vi "Stereo - Analyze Calibrated Image.vi"(8 "error in (no error)":errorcluster, 10 "Grid Images in":T4(array[cluster]), 11 "Calibrated Images in":T1[](array[typedef])) -> (0 "error out":errorcluster, 1 "Calibration OK":bool, 2 "Grid Images out":T4(array[cluster]), 3 "Calibrated Images out":T1[](array[typedef]))   [LabVIEW 2019]
doc: "Analyses the camera model to ensure that all the grids angles are at least 3 degrees apart."
uses:
  <vilib>/vision/Image Controls.llb/IMAQ Image.ctl
  <vilib>/vision/Calibration.llb/Calibration Reference Points.ctl
panel:
  # "Overview: Analyses the camera model to ensure that all the grids angles are at least 3 degrees apart."
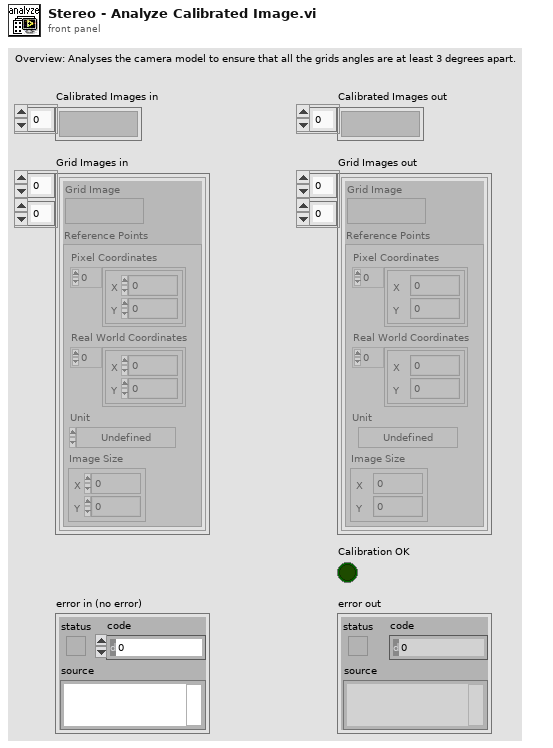
[diagram p1: front panel]
types:
  T1 = typedef "IMAQ Image.ctl" = refnum<image>
  T2 = typedef "Calibration Reference Points.ctl" = cluster{"Pixel Coordinates":cluster{"X":dbl, "Y":dbl}[], "Real World Coordinates":cluster{"X":dbl, "Y":dbl}[], "Unit":T3, "Image Size":cluster{"X":u32, "Y":u32}}
  T3 = typedef "Image Unit" = enum32{"Undefined", "Angström", "Micrometer", "Millimeter", "Centimeter", "Meter", "Kilometer", "Microinch", "Inch", "Feet", "Nautical miles", "Standard miles", "Steps"}
  T4 = cluster{"Grid Image":T1, "Reference Points":T2}[][]
  T5 = cluster{"Back Projected Points?":bool, "Undistorted Points?":bool, "Euler Angles?":bool}
  T6 = cluster{"Grid Image":T1, "Reference Points":T2}[]
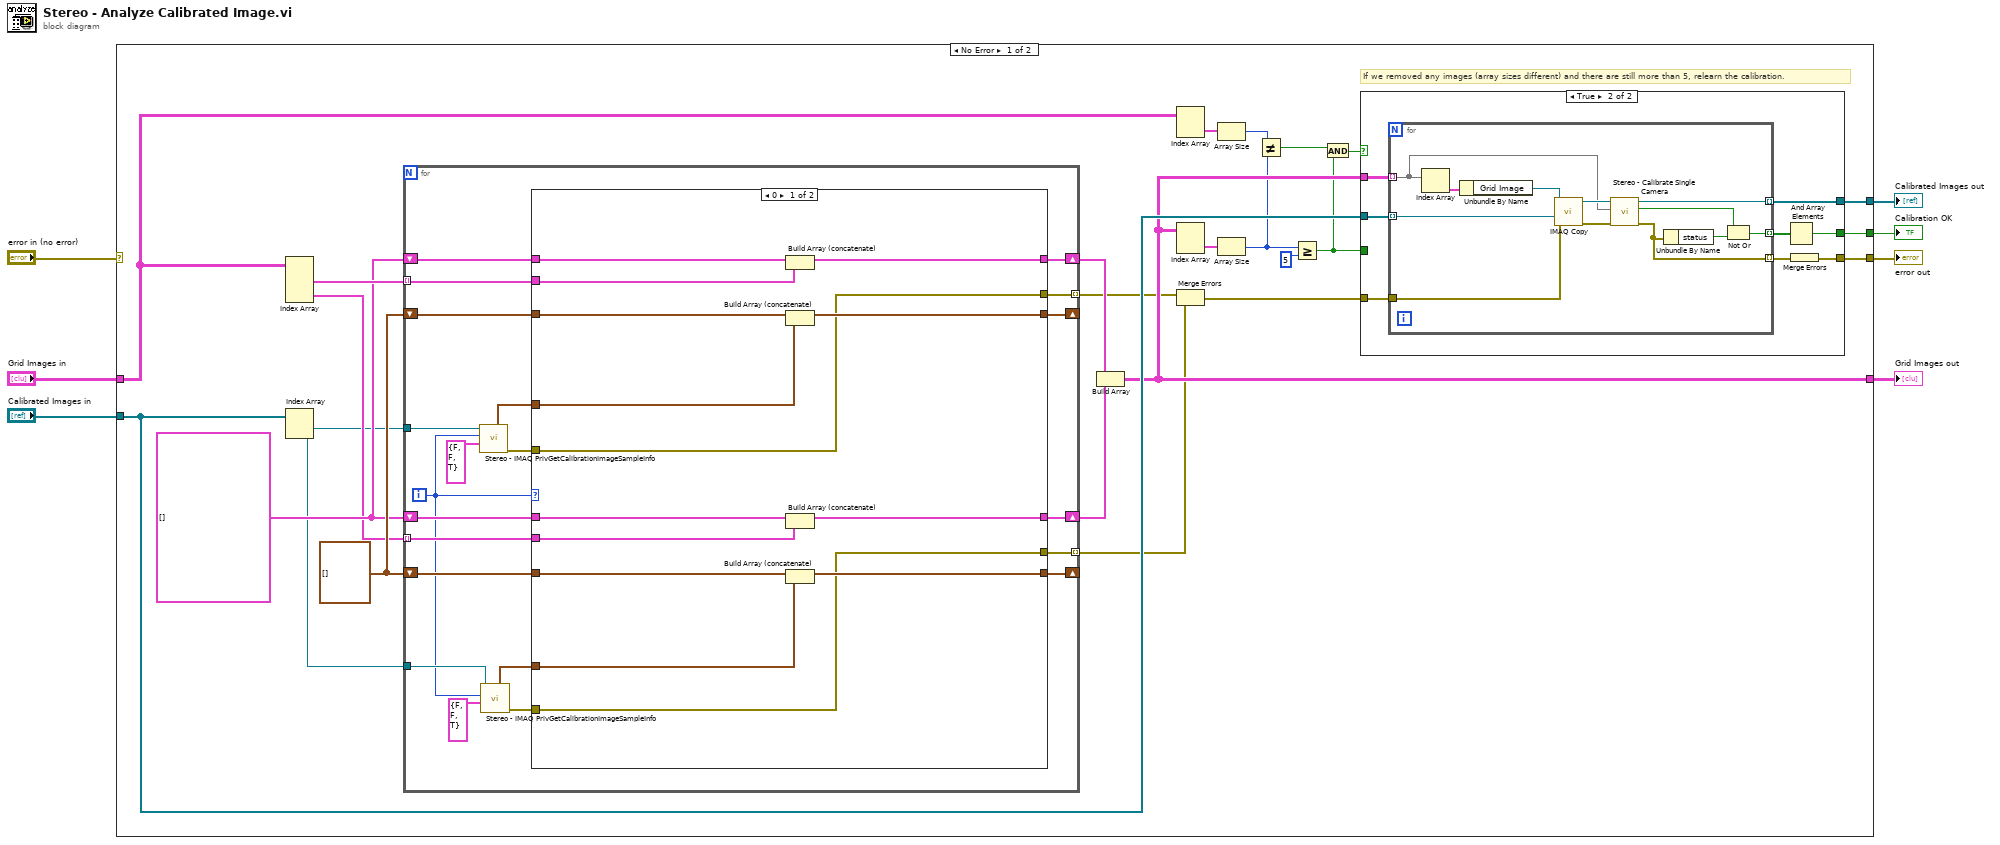
[diagram p0: block diagram]
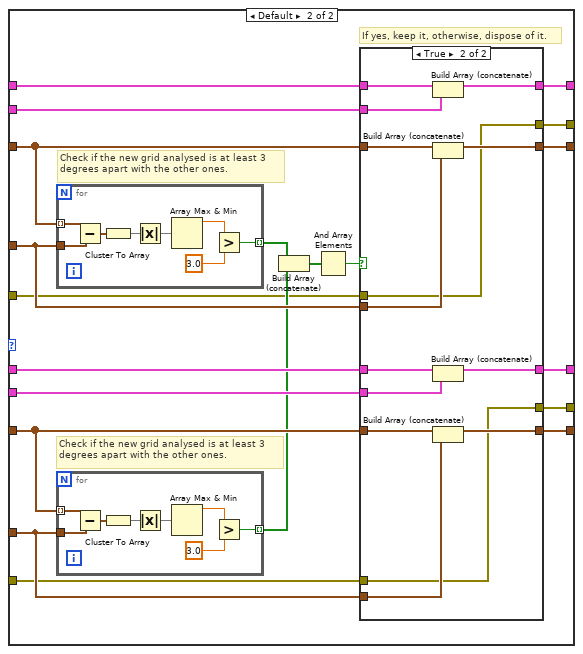
[diagram p2: hidden frame]
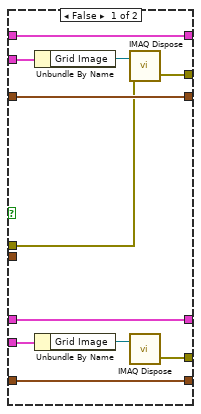
[diagram p3: hidden frame]
diagram:
  n1 = case shown="No Error" "error in (no error)" {
    selector: "error in (no error)" -> [_ w152]
    tunnel: "Calibrated Images in" -> [w32 w153]
    tunnel: "Grid Images in" -> [w31 w154]
    tunnel: [w30 w153] -> w5
    tunnel: [w29 _] -> w4
    tunnel: [w28 w154] -> w3
    tunnel: [w27 w152] -> w1
    frame No Error {
      w16 = T6 [] ("Grid Images in")
      w17 = cluster{"X":dbl, "Y":dbl, "Z":dbl}[] []
      # "If we removed any images (array sizes different) and there are still more than 5, relearn the calibration."
      n2 = Index Array(array=w31) -> (element #1=w18:T6, element #2=w15:T6)  [unwired: 4 in]
      n3 = Index Array(array=w32) -> (element #1=w14:T1, element #2=w13:T1)  [unwired: 2 in]
      n4 = for {
        shift-right: [w48] -> _
        shift-left: w17 -> [w49]
        shift-right: [w50] -> w11
        shift-left: w16 -> [w51]
        tunnel: w18 -> [w52] mode=indexing
        shift-right: [w44] -> w12
        shift-left: w16 -> [w46]
        shift-right: [w43] -> _
        shift-left: w17 -> [w47]
        tunnel: w15 -> [w45] mode=indexing
        tunnel: w14 -> [w42]
        tunnel: w13 -> [w41]
        tunnel: [w35] -> w10 mode=indexing
        tunnel: [w34] -> w9 mode=indexing
        i -> [w40]
        n5 = call "Stereo - IMAQ PrivGetCalibrationImageSampleInfo.vi"("Options"=T5 {"Back Projected Points?"=FALSE, "Undistorted Points?"=FALSE, "Euler Angles?"=TRUE}, "Index"=w40, "Template Image"=w42) -> ("error out"=w36:errorcluster, "Euler Angles"=w53:cluster{"X":dbl, "Y":dbl, "Z":dbl})  [unwired: 1 in, 6 out]
        n6 = call "Stereo - IMAQ PrivGetCalibrationImageSampleInfo.vi"("Options"=T5 {"Back Projected Points?"=FALSE, "Undistorted Points?"=FALSE, "Euler Angles?"=TRUE}, "Index"=w40, "Template Image"=w41) -> ("error out"=w33:errorcluster, "Euler Angles"=w39:cluster{"X":dbl, "Y":dbl, "Z":dbl})  [unwired: 1 in, 6 out]
        n7 = case shown="0" w40 {
          tunnel: w53 -> [w66 w85]
          tunnel: w52 -> [w64 w81]
          tunnel: w51 -> [w65 w84]
          tunnel: [w63 w82] -> w50
          tunnel: w49 -> [w67 w86]
          tunnel: [w62 w83] -> w48
          tunnel: w47 -> [w61 w74]
          tunnel: w46 -> [w60 w78]
          tunnel: w45 -> [w59 w77]
          tunnel: [w58 w76] -> w44
          tunnel: [w57 w75] -> w43
          tunnel: w39 -> [w56 w73]
          tunnel: w36 -> [w55 w71]
          tunnel: [w55 w70] -> w35
          tunnel: [w54 w69] -> w34
          tunnel: w33 -> [w54 w68]
          frame 0 {
            n8 = Build Array (concatenate)(w65, w64) -> (w63:T6)
            n9 = Build Array (concatenate)(w67, w66) -> (w62:cluster{"X":dbl, "Y":dbl, "Z":dbl}[])
            n10 = Build Array (concatenate)(w60, w59) -> (w58:T6)
            n11 = Build Array (concatenate)(w61, w56) -> (w57:cluster{"X":dbl, "Y":dbl, "Z":dbl}[])
          }
          frame Default {
            # "If yes, keep it, otherwise, dispose of it."
            # "Check if the new grid analysed is at least 3 degrees apart with the other ones."
            # "Check if the new grid analysed is at least 3 degrees apart with the other ones."
            n12 = for {
              tunnel: w86 -> [w128] mode=indexing
              tunnel: w85 -> [w124]
              tunnel: [w123] -> w80 mode=indexing
              n13 = Subtract(x=w128, y=w124) -> (x-y=w127:cluster{"X":dbl, "Y":dbl, "Z":dbl})
              n14 = Cluster To Array(cluster=w127) -> (array=w122:dbl[])
              n15 = Absolute Value(x=w122) -> (abs(x)=w121:dbl[])
              n16 = Array Max & Min(array=w121) -> (max value=w126:dbl)  [unwired: 3 out]
              n17 = Greater?(x=w126, y=3.0) -> (0:w123:bool)
            }
            n18 = for {
              tunnel: w74 -> [w95] mode=indexing
              tunnel: w73 -> [w91]
              tunnel: [w90] -> w72 mode=indexing
              n19 = Subtract(x=w95, y=w91) -> (x-y=w94:cluster{"X":dbl, "Y":dbl, "Z":dbl})
              n20 = Cluster To Array(cluster=w94) -> (array=w89:dbl[])
              n21 = Absolute Value(x=w89) -> (abs(x)=w88:dbl[])
              n22 = Array Max & Min(array=w88) -> (max value=w93:dbl)  [unwired: 3 out]
              n23 = Greater?(x=w93, y=3.0) -> (0:w90:bool)
            }
            n24 = Build Array (concatenate)(w80, w72) -> (w79:bool[])
            n25 = And Array Elements(Boolean array=w79) -> (logical AND=w87:bool)
            n26 = case shown="True" w87 {
              tunnel: w81 -> [w104 w120]
              tunnel: w84 -> [w106 w119]
              tunnel: [w106 w118] -> w82
              tunnel: w85 -> [_ w117]
              tunnel: w86 -> [w105 w116]
              tunnel: [w105 w115] -> w83
              tunnel: w78 -> [w99 w114]
              tunnel: w77 -> [w100 w113]
              tunnel: [w99 w112] -> w76
              tunnel: w74 -> [w102 w111]
              tunnel: w73 -> [_ w110]
              tunnel: [w102 w109] -> w75
              tunnel: w71 -> [w98 w108]
              tunnel: [w97 w108] -> w70
              tunnel: [w96 w107] -> w69
              tunnel: w68 -> [_ w107]
              frame False {
                n27 = Unbundle By Name(w104) -> ("Grid Image"=w103:T1)
                n28 = Unbundle By Name(w100) -> ("Grid Image"=w101:T1)
                n29 = call "IMAQ Dispose"("Image"=w103, "error in (no error)"=w98) -> ("error out"=w97:errorcluster)  [unwired: 1 in, 3 out]
                n30 = call "IMAQ Dispose"("Image"=w101) -> ("error out"=w96:errorcluster)  [unwired: 2 in, 3 out]
              }
              frame True {
                n31 = Build Array (concatenate)(w119, w120) -> (w118:T6)
                n32 = Build Array (concatenate)(w116, w117) -> (w115:cluster{"X":dbl, "Y":dbl, "Z":dbl}[])
                n33 = Build Array (concatenate)(w114, w113) -> (w112:T6)
                n34 = Build Array (concatenate)(w111, w110) -> (w109:cluster{"X":dbl, "Y":dbl, "Z":dbl}[])
              }
            }
          }
        }
      }
      n35 = Build Array(w11, w12) -> (w28:T4)
      n36 = Index Array(array=w31) -> (element=w21:T6)  [unwired: 2 in]
      n37 = Index Array(array=w28) -> (element=w22:T6)  [unwired: 2 in]
      n38 = Merge Errors(w10, w9) -> (w8:errorcluster)
      n39 = Array Size(array=w21) -> (size(s)=w20:i32)
      n40 = Array Size(array=w22) -> (size(s)=w24:i32)
      n41 = Not Equal?(x=w20, y=w24) -> (x != y?=w23:bool)
      n42 = Greater Or Equal?(x=w24, y=5) -> (x >= y?=w19:bool)
      n43 = And(x=w23, y=w19) -> (x .and. y?=w26:bool)
      n44 = case shown="True" w26 {
        tunnel: w28 -> [_ w139]
        tunnel: [w131 w138] -> w30
        tunnel: [w130 w135] -> w29
        tunnel: w32 -> [w131 w137]
        tunnel: w19 -> [w130 _]
        tunnel: [w129 w133] -> w27
        tunnel: w8 -> [w129 w132]
        frame False {
        }
        frame True {
          n45 = for {
            tunnel: w137 -> [w149] mode=indexing
            tunnel: w139 -> [w144] mode=indexing
            tunnel: [w142] -> w138 mode=indexing
            tunnel: [w147] -> w136 mode=indexing
            tunnel: [w141] -> w134 mode=indexing
            tunnel: w132 -> [w140]
            n46 = Index Array(array=w144) -> (element=w151:cluster{"Grid Image":T1, "Reference Points":T2})  [unwired: 1 in]
            n47 = Unbundle By Name(w151) -> ("Grid Image"=w150:T1)
            n48 = call "IMAQ Copy"("error in (no error)"=w140, "Image Dst"=w149, "Image Src"=w150) -> ("error out"=w145:errorcluster, "Image Dst Out"=w146:T1)  [unwired: 3 out]
            n49 = call "Stereo - Calibrate Single Camera.vi"("error in (no error)"=w145, "Calibration Grids"=w144, "Image in"=w146) -> ("error out"=w141:errorcluster, "Insufficient Data"=w143:bool, "Image out"=w142:T1)  [unwired: 6 out]
            n50 = Unbundle By Name(w141) -> ("status"=w148:bool)
            n51 = Not Or(1:w148, 2:w143) -> (0:w147:bool)
          }
          n52 = And Array Elements(Boolean array=w136) -> (logical AND=w135:bool)
          n53 = Merge Errors(w134) -> (w133:errorcluster)
        }
      }
    }
    frame Error {
    }
  }
  "Calibrated Images out" <- w5
  "Calibration OK" <- w4
  "Grid Images out" <- w3
  "error out" <- w1
